vi "IDS_SubMasterExample_Discovery.vi"   [LabVIEW 2016]
types:
  T1 = cluster{"IP":string, "DeviceType":string, "SerialNumber":string, "DeviceName":string, "macAddress":string, "locked":bool}[]
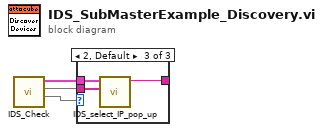
[diagram p0: block diagram]
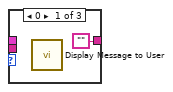
[diagram p2: hidden frame]
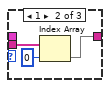
[diagram p3: hidden frame]
diagram:
  n1 = call "IDS_Check.vi"() -> (1:w1, 2:w2, "Found Devices"=w3:T1)  [unwired: 8 in, 1 out]
  n2 = case shown="2, Default" w1 {
    tunnel: w3 -> [_ _ w10]
    tunnel: w2 -> [_ w6 w9]
    tunnel: ["" w5 w8] -> _
    frame 0 {
      n3 = call "Display Message to User"() -> ()  [unwired: 10 in, 2 out]
    }
    frame 1 {
      n4 = Index Array(array=w6, index=0) -> (element=w5)
    }
    frame 2, Default {
      n5 = call "IDS_select_IP_pop_up.vi"("IPs"=w9, "Found Devices"=w10) -> ("IP"=w8:string)  [unwired: 8 in, 1 out]
    }
  }
